vi "ReadRevCtrl.vi"(2 "Device":i16=1) -> (0 "RevCTRL value":u32)   [LabVIEW 2022 SP3]
panel:
  out "error out":errorcluster
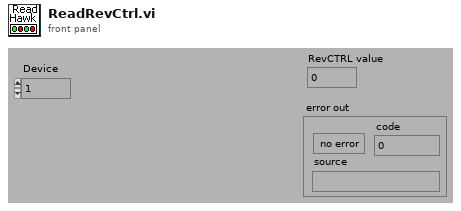
[diagram p1: front panel]
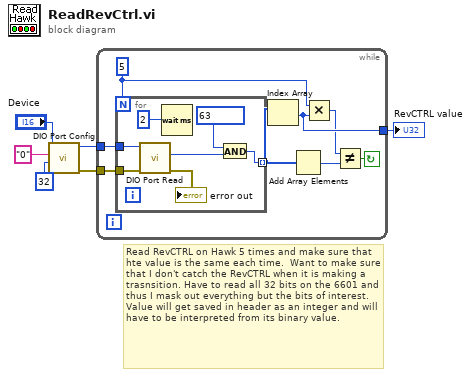
[diagram p0: block diagram]
diagram:
  # "Read RevCTRL on Hawk 5 times and make sure that hte value is the same each time.  Want to make sure that I don't catch the RevCTRL when it is making a trasnsition. Have to read all 32 bits on the 6601 and thus I mask out everything but the bits of interest. Value will get saved in header as an integer and will have to be interpreted from its binary value."
  n1 = call <vilib>:"DIO Port Config.vi"("port width"=32, "digital channel"="0", "device"="Device") -> ("error out"=w4:errorcluster, "task ID out"=w5:u32)  [unwired: 7 in]
  n2 = while {
    tunnel: w4 -> [w14]
    tunnel: w5 -> [w13]
    tunnel: [w11] -> w6
    stop <- w8 continue-if-true
    w7 = 5
    n3 = for {
      N: w7 -> [_]
      tunnel: w14 -> [w21]
      tunnel: w13 -> [w20]
      tunnel: [w15] -> w12 mode=indexing
      n4 = call <vilib>:"DIO Port Read.vi"("error in (no error)"=w21, "task ID"=w20) -> ("error out"=→"error out":errorcluster, "pattern"=w16:u32)  [unwired: 7 in, 1 out]
      n5 = Wait (ms)(milliseconds to wait=2) -> ()  [unwired: 1 out]
      n6 = And(x=63, y=w16) -> (x .and. y?=w15:u32)
    }
    n7 = Index Array(array=w12) -> (element=w11:u32)  [unwired: 1 in]
    n8 = Add Array Elements(numeric array=w12) -> (sum=w10:u32)
    n9 = Multiply(x=w7, y=w11) -> (x*y=w9:u32)
    n10 = Not Equal?(x=w9, y=w10) -> (x != y?=w8:bool)
  }
  "RevCTRL value" <- w6
